vi "Method_Const.vi"(4 "Value":i16, 5 "Value A":refnum<class "Abs_I16 Integer.lvclass">) -> (1 "Result":refnum<class "Abs_Boolean.lvclass">)   [LabVIEW 2021, in "Less Equal_I16.lvclass"]
uses:
  Less Equal_I16.lvclass
  Abs_Types/I16 Integer/Abs_I16 Integer.lvclass
  C:/Program Files (x86)/National Instruments/LabVIEW 2021/vi.lib/TSA/Abstract Data Classes/Abs_Types/Numeric/Abs_Numeric.lvclass
  Abs_Types/Boolean/Abs_Boolean.lvclass
  C:/TSA/LV_Abstract/Source/Functions/Support/Compare/Two Term/I16/AbsComp_Two Term_I16.lvclass
  C:/Program Files (x86)/National Instruments/LabVIEW 2021/vi.lib/TSA/Abstract Data Classes/Abs_Types/Boolean/Abs_Boolean.lvclass
  Support/Compare/Two Term/I16/AbsComp_Two Term_I16.lvclass/AbsComp_Two Term_I16.ctl
  Support/Compare/Two Term/I16/Properties/Write Numeric A.vi
  Support/Compare/Two Term/I16/Properties/Write Numeric B.vi
  Constants/Support/I16/Const_I16.lvclass
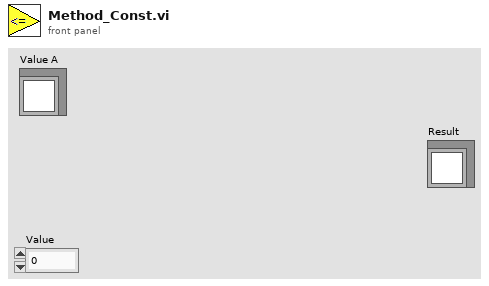
[diagram p1: front panel]
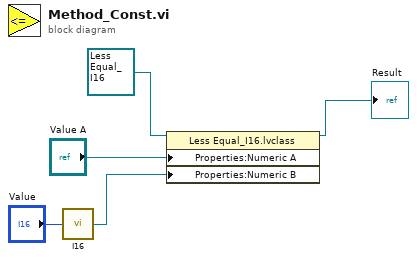
[diagram p0: block diagram]
diagram:
  n1 = call "I16.vi"("Value"="Value") -> ("Constant"=w2:refnum<class "Abs_I16 Integer.lvclass">)  [unwired: 4 in]
  n2 = property class="Less Equal_I16.lvclass"(reference=refnum<class "Less Equal_I16.lvclass"> refnum ("Greater 0_U64.lvclass"), "Properties:Numeric A"="Value A", "Properties:Numeric B"=w2) -> (reference out=→"Result":refnum<class "Less Equal_I16.lvclass">)  [unwired: 1 in, 1 out]
